vi "Resolve Linkaging.vi"(7 "Command/Response Refnum in":T2 format="%.0x", 8 "error in (no error)":errorcluster, 10 "Command/Response Format":string, 11 "Linked Channels":T1[](array[typedef]) {"Channel Refnum" format="%.0x"}) -> (0 "error out":errorcluster, 2 "Linked Channels out":T3[](array[typedef]))   [LabVIEW 2018, in "Instrument Addon Scripting API.lvlib"]
uses:
  Instrument Addon Scripting API.lvlib
  Addon/Addon Shared/Types/Linked Channel Cluster.ctl
  <vilib>/NI Veristand/Custom Device API/Custom Device Item Ref.ctl
  TypeDefs/Linked Channel.ctl
  Addon/Addon Shared/SubVIs/Constants.vi
  Addon/Addon Shared/Instrument Addon Shared.lvlib
  <vilib>/NI VeriStand/Custom Device API/Custom Device API.lvlib
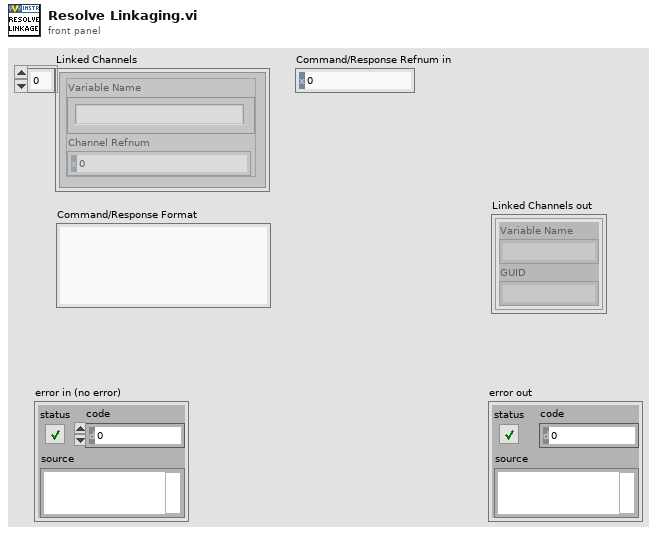
[diagram p1: front panel]
types:
  T1 = typedef "Instrument Addon Scripting API.lvlib/Linked Channel.ctl" = cluster{"Variable Name":string, "Channel Refnum":T2}
  T2 = typedef "Custom Device API.lvlib/Custom Device Item Ref.ctl" = u64
  T3 = typedef "Instrument Addon Shared.lvlib/Linked Channel Cluster.ctl" = cluster{"Variable Name":string, "GUID":string}
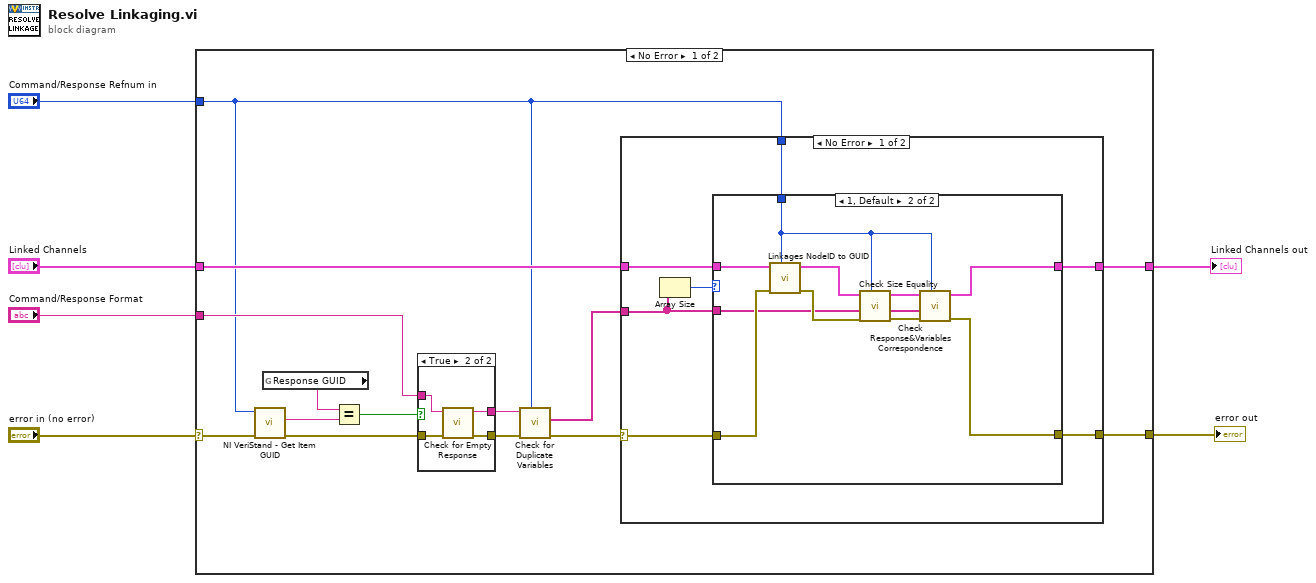
[diagram p0: block diagram]
diagram:
  n1 = case shown="No Error" "error in (no error)" {
    selector: "error in (no error)" -> [w11 w47]
    tunnel: [w20 w47] -> w6
    tunnel: [w19 _] -> w5
    tunnel: "Command/Response Refnum in" -> [w7 _]
    tunnel: "Linked Channels" -> [w18 _]
    tunnel: "Command/Response Format" -> [w16 _]
    frame No Error {
      n2 = call <vilib>:"NI VeriStand - Get Item GUID.vi"("error in (no error)"=w11, "Item Ref in"=w7) -> ("error out"=w12:errorcluster, "GUID"=w9:string)  [unwired: 7 in, 1 out]
      n3 = global read "Constants.vi" "Response GUID"() -> (w10:string)
      n4 = Equal?(x=w10, y=w9) -> (x = y?=w8:bool)
      n5 = case shown="True" w8 {
        tunnel: [w21 w26] -> w17
        tunnel: w16 -> [w22 w25]
        tunnel: [w22 w24] -> w15
        tunnel: w12 -> [w21 w23]
        frame False {
        }
        frame True {
          n6 = call "Check for Empty Response.vi"("Error In"=w23, "Response Format in"=w25) -> ("Error Out"=w26:errorcluster, "Response Format out"=w24:string)  [unwired: 8 in]
        }
      }
      n7 = call "Check for Duplicate Variables.vi"("Command/Response Refnum in"=w7, "error in (no error)"=w17, "Command/Response Format in"=w15) -> ("error out"=w14:errorcluster, "Variables"=w13:string[])  [unwired: 6 in, 1 out]
      n8 = case shown="No Error" w14 {
        selector: w14 -> [w28 w46]
        tunnel: [w33 w46] -> w20
        tunnel: w18 -> [w32 _]
        tunnel: w13 -> [w31 _]
        tunnel: [w30 _] -> w19
        tunnel: w7 -> [w29 _]
        frame No Error {
          n9 = Array Size(array=w31) -> (size(s)=w27:i32)
          n10 = case shown="1, Default" w27 {
            tunnel: w32 -> [_ w45]
            tunnel: w28 -> [w34 w44]
            tunnel: [w34 w41] -> w33
            tunnel: w31 -> [_ w40]
            tunnel: [_ w39] -> w30
            tunnel: w29 -> [_ w35]
            frame 0 {
            }
            frame 1, Default {
              n11 = call "Linkages NodeID to GUID.vi"("Command/Response Refnum in"=w35, "error in (no error)"=w44, "Linked Channels in"=w45) -> ("error out"=w43:errorcluster, "Linked Channels out"=w42:cluster{"Variable Name":string, "GUID":string}[])  [unwired: 7 in]
              n12 = call "Check Size Equality.vi"("Command/Response Refnum in"=w35, "Error In"=w43, "Variables"=w40, "Linked Channels in"=w42) -> ("Error Out"=w38:errorcluster, "Variables out"=w36:string[], "Linked Channels out"=w37:cluster{"Variable Name":string, "GUID":string}[])  [unwired: 5 in]
              n13 = call "Check Response&Variables Correspondence.vi"("Command/Response Refnum in"=w35, "error in (no error)"=w38, "Variables in"=w36, "Linked Channels in"=w37) -> ("error out"=w41:errorcluster, "Linked Channels out"=w39:T3[])  [unwired: 6 in]
            }
          }
        }
        frame Error {
        }
      }
    }
    frame Error {
    }
  }
  "error out" <- w6
  "Linked Channels out" <- w5
